vi "validate receive package.vi"(10 "Send package":string, 11 "Receive package":string) -> (3 "Valid receive package":bool)   [LabVIEW 2014, in "HPCNC.lvlib"]
uses:
  HPCNC.lvlib
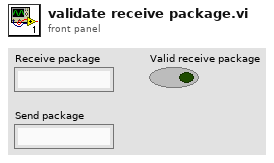
[diagram p1: front panel]
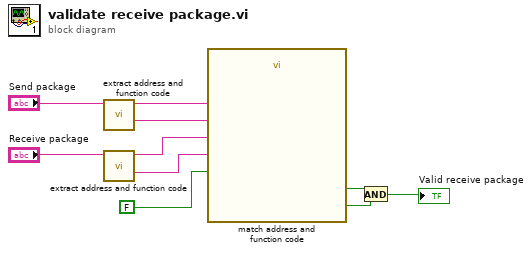
[diagram p0: block diagram]
diagram:
  n1 = call "extract address and function code.vi"("Cmd to Send"="Send package") -> ("Function Code"=w5:string, "SendAddress"=w4:string)  [unwired: 9 in]
  n2 = call "extract address and function code.vi"("Cmd to Send"="Receive package") -> ("Function Code"=w3:string, "SendAddress"=w2:string)  [unwired: 9 in]
  n3 = call "match address and function code.vi"("Address"=w4, "Received Address"=w2, "Received Function Code"=w3, "Function Code"=w5, "NewCmd"=FALSE) -> ("Address?"=w7:bool, "FCode?"=w8:bool)  [unwired: 9 in]
  n4 = And(x=w7, y=w8) -> (x .and. y?=→"Valid receive package":bool)
